vi "Vision Processing.vi"(4 "error in (no error)":errorcluster, 7 "Image Size":T6=enum."320x240") -> ()   [LabVIEW 2014]
doc: "This VI runs in parallel to other tasks. It gets images from the camera, processes them for color or shape and use that information to affect robot behavior."
uses:
  <vilib>/Rock Robotics/WPI/Camera/WPI_CameraImageSize.ctl
  Program Files (x86)/National Instruments/LabVIEW 2014/examples/FRC/roboRIO/Vision/2015 Vision Example/Vision Support Code/Camera Types.ctl
  <vilib>/Rock Robotics/WPI/Camera/WPI_CameraWhite Balance Values.ctl
  <vilib>/Rock Robotics/WPI/Camera/WPI_CameraExposure Values.ctl
  <vilib>/Rock Robotics/WPI/Camera/WPI_CameraFrameRate.ctl
  <vilib>/vision/Pattern Matching.llb/IMAQ Match Range Setting.ctl
  <vilib>/vision/Pattern Matching.llb/IMAQ Curve Parameters.ctl
  Robot Global Data.vi
  Global 2.vi
  <vilib>/vision/NI_Vision_Development_Module.lvlib
panel:
  out "Scale":dbl
  out "LeftSide":dbl
  out "RightSide":dbl
  out "Detected Totes":T1(array[cluster]) {"Normalized Rect"."Numeric 5" format="%#_2g"; "Normalized Rect"."Numeric 3" format="%#_2g"; "Normalized Rect"."Numeric 2" format="%#_2g"; "Normalized Rect"."Numeric" format="%#_2g"}
  out "Sorted Scores":T2(array[cluster]) {"Correlation" format="%#_3g"; "Scale %" format="%#_3g"; "Score" format="%#_3g"}
  in  "Score Threshold":dbl=75.0
  in  "Annotate":bool=TRUE
  in  "Camera Type":T3=enum."MS HD3000 square"
  out "ms to process":u32
  out "Camera Image":T4(plugin-control)
  out "Template 2":T4(plugin-control)
  out "Masked":T4(plugin-control)
  in  "Tote Color":T5={"Hue"={23.67058792990901, 48.923317529462665}, "Sat"={66.78571428571429, 255.0}, "Val"={48.571428571428584, 255.0}} {"Hue" scale=0.0..255.0 scale format="%#_3g"}
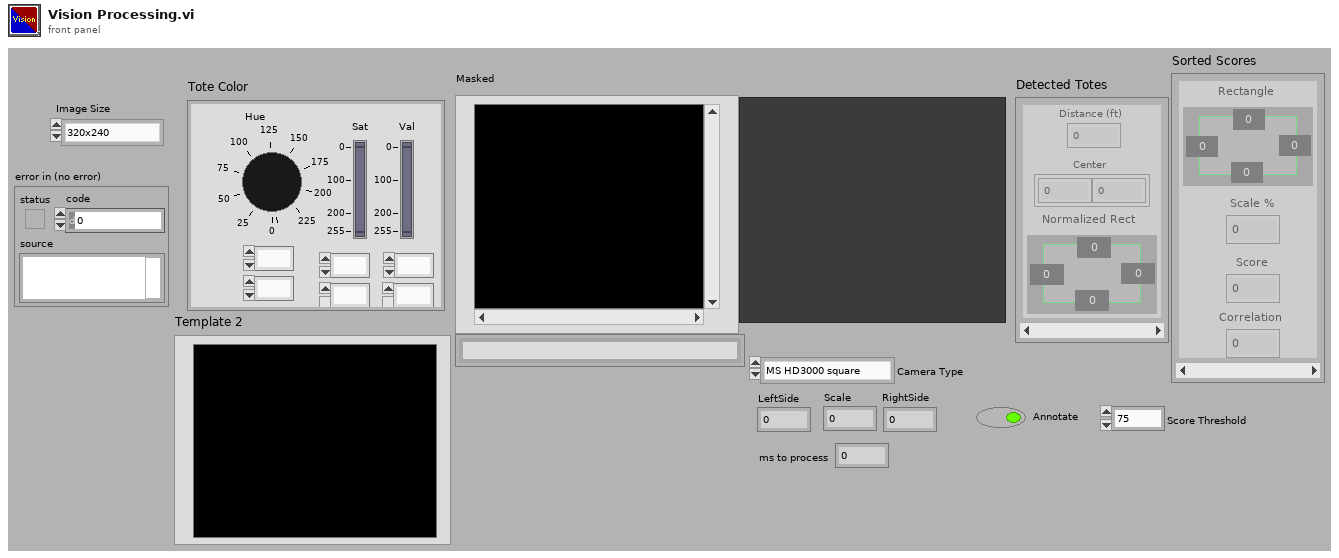
[diagram p1: front panel]
types:
  T1 = cluster{"Distance (ft)":dbl, "Center":cluster{dbl, dbl}, "Normalized Rect":cluster{"Numeric":dbl, "Numeric 2":dbl, "Numeric 3":dbl, "Numeric 5":dbl}}[]
  T2 = cluster{"Rectangle":cluster{"Numeric":dbl, "Numeric 2":dbl, "Numeric 3":dbl, "Numeric 5":dbl}, "Scale %":dbl, "Score":dbl, "Correlation":dbl}[]
  T3 = typedef "Camera Types.ctl" = enum16{"206", "1011", "1013", "MS HD3000 square", "MS HD3000 640x480"}
  T4 = typedef "IMAQ Image.ctl" = refnum<image>
  T5 = cluster{"Hue":cluster{dbl, dbl}, "Sat":cluster{dbl, dbl}, "Val":cluster{dbl, dbl}}
  T6 = typedef "WPI_CameraImageSize.ctl" = enum16{"640x480", "320x240", "160x120", "Custom"}
  T7 = cluster{"Rotation":bool, "Scale":bool, "Occlusion":bool, "Reserved":bool, "Reserved":bool, "Reserved":bool}
  T8 = typedef "IMAQ Curve Parameters.ctl" = cluster{"Extraction Mode":u32, "Edge Threshold":i32, "Edge Filter Size":u32, "Min Length":i32, "Row Search Step Size":i32, "Col Search Step Size":i32, "Max Endpoint Gap":i32, "Closed":bool, "Subpixel":bool}
  T9 = typedef "IMAQ Match Range Setting.ctl" = cluster{"Match Constraints":u32, "Min":dbl, "Max":dbl}
  T10 = typedef "Image Type" = u32
  T11 = typedef "Particle Parameters" = i32
  T12 = typedef "WPI_CameraFrameRate.ctl" = u32
  T13 = typedef "WPI_CameraExposure Values.ctl" = enum16{"Auto", "Flicker-free 50 Hz", "Flicker-free 60 Hz", "Hold current", "Custom"}
  T14 = typedef "WPI_CameraWhite Balance Values.ctl" = enum16{"Auto", "Fixed indoor", "Fixed outdoor 1", "Fixed outdoor 2", "Fixed fluorescent 1", "Fixed fluorescent 2", "Hold current", "Custom"}
  T15 = typedef "WPI_CameraDevRef.ctl" = cluster{"Camera Address":string, "CameraStatus":errorcluster}
  T16 = cluster{"[0]":dbl, "[1]":dbl, "[2]":dbl, "[3]":dbl}
  T17 = cluster{"[0]":dbl, "[1]":dbl, "[2]":dbl, "[3]":dbl, "[4]":dbl}
  T18 = typedef "ROI Descriptor" = cluster{"Global Rectangle":i32[], "Contours":cluster{"ID":enum32{"External", "Internal"}, "Type":u32, "Coordinates":i32[]}[]}
  T19 = typedef "IMAQ GM Match Report.ctl" = cluster{"Position":cluster{"x":sgl, "y":sgl}, "Angle":sgl, "Scale":sgl, "Score":sgl, "Bounding Box":cluster{"x":sgl, "y":sgl}[], "Contrast Reversed":bool, "Occlusion %":sgl, "Template Target Curve Score":sgl, "Target Template Curve Score":sgl, "Correlation Score":sgl}
  T20 = cluster{cluster{"[0]":dbl, "[1]":dbl, "[2]":dbl, "[3]":dbl}, "Position":cluster{"x":sgl, "y":sgl}, "Bounding Box":cluster{"x":sgl, "y":sgl}[], "Scale":sgl, "Score":sgl, "Correlation Score":sgl}
  T21 = cluster{"Rectangle":cluster{"Numeric":dbl, "Numeric 2":dbl, "Numeric 3":dbl, "Numeric 5":dbl}, "Scale":dbl, "Score":dbl, "Correlation":dbl}[]
  T22 = cluster{"Sorted Scores[0]":cluster{"Rectangle":cluster{"Numeric":dbl, "Numeric 2":dbl, "Numeric 3":dbl, "Numeric 5":dbl}, "Scale":dbl, "Score":dbl, "Correlation":dbl}, "Sorted Scores[1]":cluster{"Rectangle":cluster{"Numeric":dbl, "Numeric 2":dbl, "Numeric 3":dbl, "Numeric 5":dbl}, "Scale":dbl, "Score":dbl, "Correlation":dbl}, "Sorted Scores[2]":cluster{"Rectangle":cluster{"Numeric":dbl, "Numeric 2":dbl, "Numeric 3":dbl, "Numeric 5":dbl}, "Scale":dbl, "Score":dbl, "Correlation":dbl}, "Sorted Scores[3]":cluster{"Rectangle":cluster{"Numeric":dbl, "Numeric 2":dbl, "Numeric 3":dbl, "Numeric 5":dbl}, "Scale":dbl, "Score":dbl, "Correlation":dbl}, "Sorted Scores[4]":cluster{"Rectangle":cluster{"Numeric":dbl, "Numeric 2":dbl, "Numeric 3":dbl, "Numeric 5":dbl}, "Scale":dbl, "Score":dbl, "Correlation":dbl}, "Sorted Scores[5]":cluster{"Rectangle":cluster{"Numeric":dbl, "Numeric 2":dbl, "Numeric 3":dbl, "Numeric 5":dbl}, "Scale":dbl, "Score":dbl, "Correlation":dbl}, "Sorted Scores[6]":cluster{"Rectangle":cluster{"Numeric":dbl, "Numeric 2":dbl, "Numeric 3":dbl, "Numeric 5":dbl}, "Scale":dbl, "Score":dbl, "Correlation":dbl}, "Sorted Scores[7]":cluster{"Rectangle":cluster{"Numeric":dbl, "Numeric 2":dbl, "Numeric 3":dbl, "Numeric 5":dbl}, "Scale":dbl, "Score":dbl, "Correlation":dbl}, "Sorted Scores[8]":cluster{"Rectangle":cluster{"Numeric":dbl, "Numeric 2":dbl, "Numeric 3":dbl, "Numeric 5":dbl}, "Scale":dbl, "Score":dbl, "Correlation":dbl}}
  T23 = cluster{"Rectangle":cluster{"Numeric":dbl, "Numeric 2":dbl, "Numeric 3":dbl, "Numeric 5":dbl}, "Scale":dbl, "Score":dbl, "Correlation":dbl}
  T24 = cluster{"Numeric":dbl, "Numeric 2":dbl, "Numeric 3":dbl, "Numeric 5":dbl}
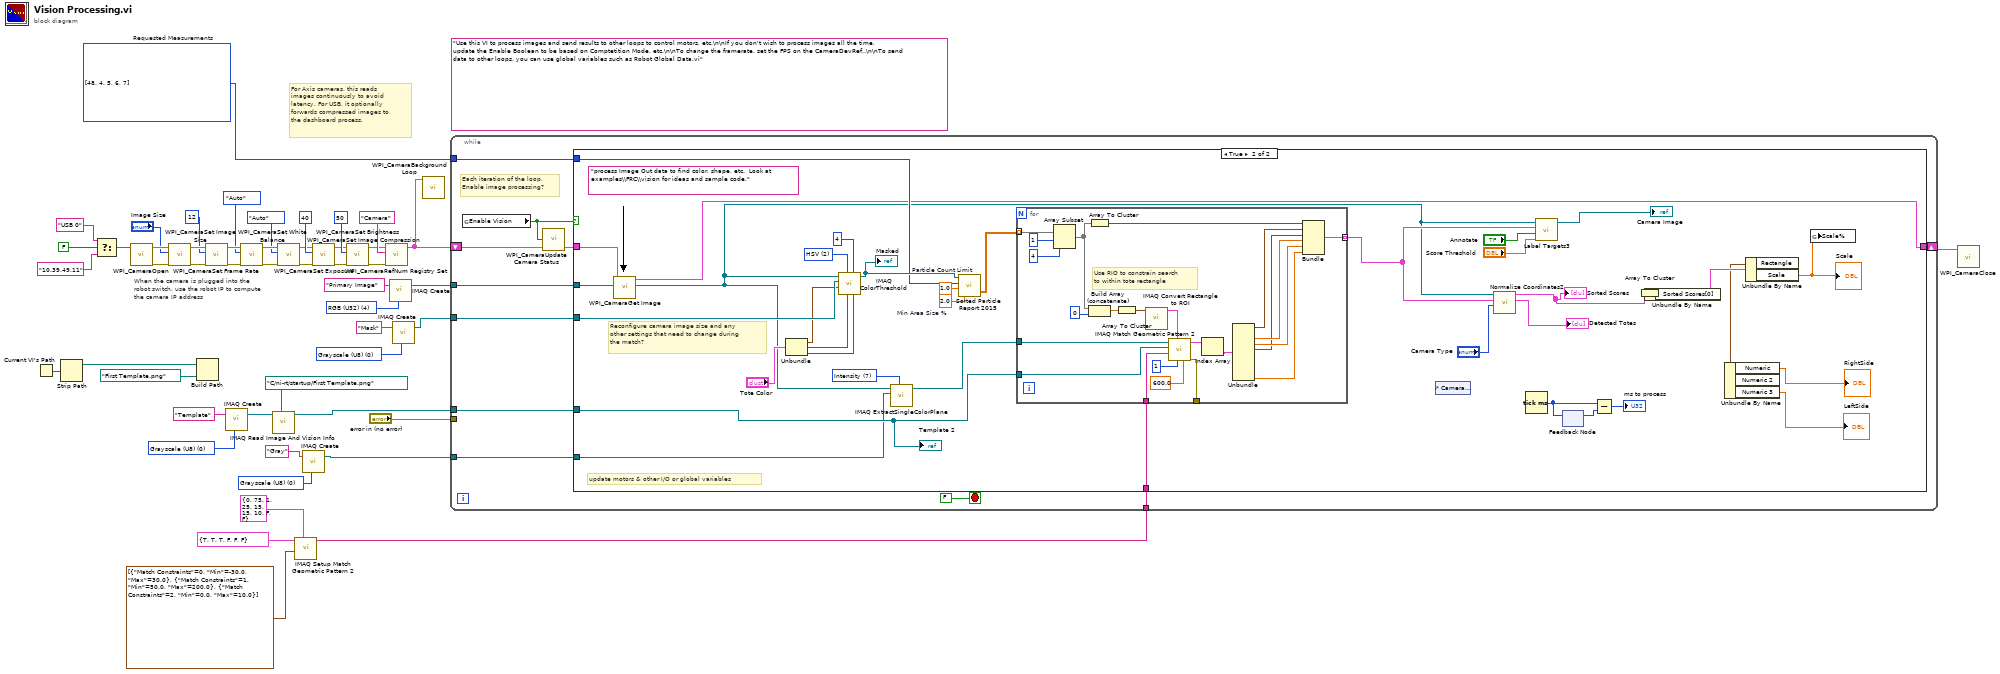
[diagram p0: block diagram]
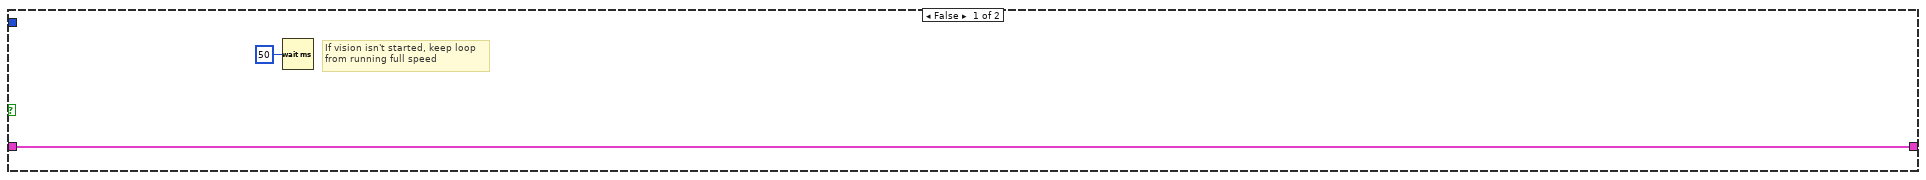
[diagram p2: hidden frame]
diagram:
  w11 = T10 0 items=["Grayscale (U8)", "Grayscale (I16)", "Grayscale (SGL)", "Complex (CSG)", "RGB (U32)", "HSL (U32)", "RGB (U64)", "Grayscale (U16)"] ("Image Type")
  w15 = T10 0 items=["Grayscale (U8)", "Grayscale (I16)", "Grayscale (SGL)", "Complex (CSG)", "RGB (U32)", "HSL (U32)", "RGB (U64)", "Grayscale (U16)"] ("Image Type")
  w16 = T11[] [48, 4, 5, 6, 7] items=["Center of Mass X", "Center of Mass Y", "First Pixel X", "First Pixel Y", "Bounding Rect Left", "Bounding Rect Top", "Bounding Rect Right", "Bounding Rect Bottom", "Max Feret Diameter Start X", "Max Feret Diameter Start Y", "Max Feret Diameter End X", "Max Feret Diameter End Y", "Max Horiz. Segment Length Left", "Max Horiz. Segment Length Right", "Max Horiz. Segment Length Row", "-", "Bounding Rect Width", "Bounding Rect Height", "Bounding Rect Diagonal", "Perimeter", "Convex Hull Perimeter", "Holes' Perimeter", "Max Feret Diameter", "Equivalent Ellipse Major Axis", "Equivalent Ellipse Minor Axis", "Equivalent Ellipse Minor Axis (Feret)", "Equivalent Rect Long Side", "Equivalent Rect Short Side", "Equivalent Rect Diagonal", "Equivalent Rect Short Side (Feret)", "Average Horiz. Segment Length", "Average Vert. Segment Length", "Hydraulic Radius", "Waddel Disk Diameter", "-", "Area", "Holes' Area", "Particle & Holes' Area", "Convex Hull Area", "Image Area", "-", "Number of Holes", "Number of Horiz. Segments", "Number of Vert. Segments", "-", "Orientation", "Max Feret Diameter Orientation", "-", "% Area/Image Area", "% Area/(Particle & Holes' Area)", "Ratio of Equivalent Ellipse Axes", "Ratio of Equivalent Rect Sides", "-", "Elongation Factor", "Compactness Factor", "Heywood Circularity Factor", "Type Factor", "-", "Sum X", "Sum Y", "Sum XX", "Sum XY", "Sum YY", "Sum XXX", "Sum XXY", "Sum XYY", "Sum YYY", "-", "Moment of Inertia XX", "Moment of Inertia XY", "Moment of Inertia YY", "Moment of Inertia XXX", "Moment of Inertia XXY", "Moment of Inertia XYY", "Moment of Inertia YYY", "Norm. Moment of Inertia XX", "Norm. Moment of Inertia XY", "Norm. Moment of Inertia YY", "Norm. Moment of Inertia XXX", "Norm. Moment of Inertia XXY", "Norm. Moment of Inertia XYY", "Norm. Moment of Inertia YYY", "Hu Moment 1", "Hu Moment 2", "Hu Moment 3", "Hu Moment 4", "Hu Moment 5", "Hu Moment 6", "Hu Moment 7"]  # Requested Measurements
  w19 = T10 0 items=["Grayscale (U8)", "Grayscale (I16)", "Grayscale (SGL)", "Complex (CSG)", "RGB (U32)", "HSL (U32)", "RGB (U64)", "Grayscale (U16)"] ("Image Type")
  (unwired) "Use this VI to process images and send results to other loops to control motors, etc.\n\nIf you don't wish to process images all the time, update the Enable Boolean to be based on Comptetition Mode, etc.\n\nTo change the framerate, set the FPS on the CameraDevRef..\n\nTo send data to other loops, you can use global variables such as Robot Global Data.vi"
  w50 = T10 4 items=["Grayscale (U8)", "Grayscale (I16)", "Grayscale (SGL)", "Complex (CSG)", "RGB (U32)", "HSL (U32)", "RGB (U64)"] ("Image Type")
  # "When the camera is plugged into the\nrobot switch, use the robot IP to compute\nthe camera IP address"
  # "For Axis cameras, this reads\nimages continuously to avoid\nlatency. For USB, it optionally\nforwards compressed images to\nthe dashboard process."
  n1 = Current VI's Path() -> (path=w3:path)
  n2 = Strip Path(path=w3) -> (stripped path=w2:path)  [unwired: 1 out]
  n3 = Select(t="USB 0" ("format string"), s=FALSE ("dot notation? (F)"), f="10.39.49.11" ("format string")) -> (s? t:f=w21:string)
  n4 = call <vilib>:"WPI_CameraOpen.vi"("Camera Address"=w21) -> ("error out"=w38:errorcluster, "CameraDevRef"=w39:T15)  [unwired: 1 in, 8 out]
  n5 = call <vilib>:"WPI_CameraSet Image Size.vi"("error in (no error)"=w38, "Image Size"="Image Size", "CameraDevRef"=w39) -> ("error out"=w37:errorcluster, "CameraDevRef Out"=w40:T15)  [unwired: 1 in, 6 out]
  n6 = Build Path(base path=w2, name or relative path=path "First Template.png") -> ()  [unwired: 1 out]
  n7 = call <vilib>:"WPI_CameraSet Frame Rate.vi"("error in (no error)"=w37, "Frame Rate (fps)"=T12 12, "CameraDevRef"=w40) -> ("error out"=w36:errorcluster, "CameraDevRef Out"=w42:T15)  [unwired: 7 out]
  n8 = call "IMAQ Create"("Image Name"="Template", "Image Type"=w15) -> ("New Image"=w13:T4)  [unwired: 2 in, 2 out]
  n9 = call <vilib>:"WPI_CameraSet White Balance.vi"("error in (no error)"=w36, "White Balance"=WPI_CameraWhite_Balance_Values."Auto", "CameraDevRef"=w42) -> ("error out"=w35:errorcluster, "CameraDevRef Out"=w41:T15)  [unwired: 1 in, 6 out]
  n10 = call "IMAQ Read Image And Vision Info"("File Path"=path "C:/ni-rt/startup/First Template.png", "Image"=w13) -> ("Image Out"=w12:T4)  [unwired: 2 in, 7 out]
  n11 = call <vilib>:"WPI_CameraSet Exposure.vi"("error in (no error)"=w35, "Exposure"=WPI_CameraExposure_Values."Auto", "CameraDevRef"=w41) -> ("error out"=w34:errorcluster, "CameraDevRef Out"=w44:T15)  [unwired: 1 in, 6 out]
  n12 = call "IMAQ Setup Match Geometric Pattern 2"("Curve Parameters"=T8 {"Extraction Mode"=0, "Edge Threshold"=75, "Edge Filter Size"=1, "Min Length"=25, "Row Search Step Size"=15, "Col Search Step Size"=15, "Max Endpoint Gap"=10, "Closed"=FALSE, "Subpixel"=FALSE}, "Range Settings"=T9[] [{"Match Constraints"=0, "Min"=-30.0, "Max"=30.0}, {"Match Constraints"=1, "Min"=50.0, "Max"=200.0}, {"Match Constraints"=2, "Min"=0.0, "Max"=10.0}], "Match Mode"=T7 {"Rotation"=TRUE, "Scale"=TRUE, "Occlusion"=TRUE, "Reserved"=FALSE, "Reserved"=FALSE, "Reserved"=FALSE}) -> ("Match Geometric Pattern 2 Setup Data"=w5:string)  [unwired: 7 in, 1 out]
  n13 = call "IMAQ Create"("Image Name"="Gray", "Image Type"=w11) -> ("New Image"=w9:T4)  [unwired: 2 in, 2 out]
  n14 = call <vilib>:"WPI_CameraSet Image Compression.vi"("error in (no error)"=w34, "Compression"=40, "CameraDevRef"=w44) -> ("error out"=w33:errorcluster, "CameraDevRef Out"=w43:T15)  [unwired: 7 out]
  n15 = call <vilib>:"WPI_CameraSet Brightness.vi"("error in (no error)"=w33, "Brightness"=50, "CameraDevRef"=w43) -> ("error out"=w31:errorcluster, "CameraDevRef Out"=w32:T15)  [unwired: 7 out]
  n16 = call <vilib>:"WPI_CameraRefNum Registry Set.vi"("error in (no error)"=w31, "refnum name"="Camera", "CameraDevRef"=w32) -> ("CameraDevRef"=w27:T15)  [unwired: 8 out]
  n17 = call "IMAQ Create"("Image Name"="Primary Image", "Image Type"=w50) -> ("New Image"=w48:T4)  [unwired: 2 in, 2 out]
  n18 = call "IMAQ Create"("Image Name"="Mask", "Image Type"=w19) -> ("New Image"=w17:T4)  [unwired: 2 in, 2 out]
  n19 = call <vilib>:"WPI_CameraBackground Loop.vi"("CameraDevRef"=w27) -> ()  [unwired: 11 in]
  n20 = while {
    shift-right: [w51] -> w25
    shift-left: w27 -> [w59]
    tunnel: w48 -> [w60]
    tunnel: "error in (no error)" -> [_]
    tunnel: w17 -> [w56]
    tunnel: w16 -> [w55]
    tunnel: w12 -> [w54]
    tunnel: w9 -> [w53]
    tunnel: w5 -> [w52]
    stop <- FALSE stop-if-true
    # "Each iteration of the loop,\nEnable image processing?"
    n21 = global read "Robot Global Data.vi" "Enable Vision"() -> (w57:bool)
    n22 = call <vilib>:"WPI_CameraUpdate Camera Status.vi"("CameraDevRef In"=w59, "Enable Vision"=w57) -> ("CameraDevRef Out"=w58:T15)  [unwired: 3 in]
    n23 = case shown="True" w57 {
      tunnel: w60 -> [_ w100]
      tunnel: w58 -> [w62 w99]
      tunnel: w56 -> [_ w98]
      tunnel: w55 -> [_ w90]
      tunnel: w54 -> [_ w84]
      tunnel: w53 -> [_ w83]
      tunnel: w52 -> [_ w82]
      tunnel: [w62 w68] -> w51
      frame False {
        # "If vision isn't started, keep loop\nfrom running full speed"
        n24 = Wait (ms)(milliseconds to wait=u32 50) -> ()  [unwired: 1 out]
      }
      frame True {
        w86 = 7 items=["Red", "Green", "Blue", "Hue", "Saturation", "Luminance", "Value", "Intensity"] ("Color Plane")
        w88 = 2.0  # Min Area Size %
        w89 = 1.0  # Particle Count Limit
        w93 = u16 2 items=["RGB", "HSL", "HSV", "HSI"] ("Color Mode")
        (unwired) "process Image Out data to find color, shape, etc.  Look at examples\\FRC\\vision for ideas and sample code."
        # "update motors & other I/O or global variables"
        # "Reconfigure camera image size and any\nother settings that need to change during\nthe match?"
        n25 = call <vilib>:"WPI_CameraGet Image.vi"("Image"=w100, "CameraDevRef"=w99) -> ("Image Out"=w67:T4, "CameraDevRef Out"=w68:T15)  [unwired: 1 in, 7 out]
        n26 = Unbundle("Tote Color") -> ("Hue"=w96:cluster{dbl, dbl}, "Sat"=w95:cluster{dbl, dbl}, "Val"=w94:cluster{dbl, dbl})
        n27 = call "IMAQ ColorThreshold"("Blue or Luma or Val or Inten Range"=w94, "Replace Value"=4, "Green or Sat Range"=w95, "Color Mode"=w93, "Red or Hue Range"=w96, "Image Dst"=w98, "Image Src"=w67) -> ("Image Dst Out"=w91:T4)  [unwired: 3 in, 1 out]
        "Masked" <- w91
        n28 = call "IMAQ ExtractSingleColorPlane"("Color Plane"=w86, "Image Dst"=w83, "Image Src"=w67) -> ("Image Dst Out"=w85:T4)  [unwired: 7 in, 1 out]
        n29 = call "Sorted Particle Report 2015.vi"("Min Area Size %"=w88, "Particle Count Limit"=w89, "Pixel Measurements"=w90, "Image in"=w91) -> ("Sorted Data"=w87:dbl[][])  [unwired: 1 out]
        n30 = for {
          tunnel: w87 -> [w121] mode=indexing
          tunnel: [w120] -> w70 mode=indexing
          tunnel: w85 -> [w111]
          tunnel: w82 -> [w113]
          tunnel: w84 -> [w103]
          tunnel: [w102] -> _
          # "Use RIO to constrain search\nto within tote rectangle"
          n31 = Array Subset(array=w121, index=1, length=4) -> (w114:dbl[])
          n32 = Array To Cluster(array=w114) -> (cluster=w115:T16)
          n33 = Build Array (concatenate)(w114, 0 ("length")) -> (w118:dbl[])
          n34 = Array To Cluster(array=w118) -> (cluster=w117:T17)
          n35 = call "IMAQ Convert Rectangle to ROI"("Rectangle"=w117) -> ("ROI Descriptor"=w116:T18)  [unwired: 8 in, 1 out]
          n36 = call "IMAQ Match Geometric Pattern 2"("Minimum Match Score"=sgl 600.0, "Number of Matches Requested"=1 ("Minimum Match Score"), "ROI Descriptor"=w116, "Match Geometric Pattern 2 Setup Data"=w113, "Template Image"=w103, "Image"=w111) -> ("error out"=w102:errorcluster, "Matches (pixel)"=w109:T19[])  [unwired: 2 in, 2 out]
          n37 = Index Array(array=w109) -> (element=w108:T19)  [unwired: 1 in]
          n38 = Unbundle(w108) -> ("Position"=w107:cluster{"x":sgl, "y":sgl}, "Scale"=w106:sgl, "Score"=w105:sgl, "Bounding Box"=w101:cluster{"x":sgl, "y":sgl}[], "Correlation Score"=w104:sgl)  [unwired: 5 out]
          n39 = Bundle(w115, "Position"=w107, "Bounding Box"=w101, "Scale"=w106, "Score"=w105, "Correlation Score"=w104) -> (w120:T20)  [unwired: 1 in]
        }
        n40 = control-ref of="Camera Type"() -> ()  [unwired: 1 out]
        n41 = call "Normalize Coordinates2.vi"("Camera Type"="Camera Type", "Targets"=w70, "Image in"=w67) -> ("Found Totes"=→"Detected Totes":T1, "Sorted Scores"=w74:T21)  [unwired: 7 in]
        "Sorted Scores" <- w74
        n42 = Tick Count (ms)() -> (millisecond timer value=w80:u32)
        n43 = call "Label Targets3.vi"("Score Threshold"="Score Threshold", "Annotate"="Annotate", "Targets"=w70, "Image in"=w67) -> ("Image out"=→"Camera Image":T4)  [unwired: 7 in]
        n44 = feedback #1() -> (w81:u32)  [unwired: 1 in]
        n45 = feedback-in #1(w80) -> ()
        n46 = Subtract(x=w80, y=w81) -> (x-y=→"ms to process":u32)
        n47 = Array To Cluster(array=w74) -> (cluster=w73:T22)
        n48 = Unbundle By Name(w73) -> ("Sorted Scores[0]"=w72:T23)
        n49 = Unbundle By Name(w72) -> ("Rectangle"=w66:T24, "Scale"=w69:dbl)
        "Scale" <- w69
        n50 = Unbundle By Name(w66) -> ("Numeric"=→"RightSide":dbl, "Numeric 3"=→"LeftSide":dbl)  [unwired: 1 out]
        n51 = global write "Global 2.vi" "Scale%"(w69) -> ()
        "Template 2" <- w84
      }
    }
  }
  n52 = call <vilib>:"WPI_CameraClose.vi"("CameraDevRef"=w25) -> ()  [unwired: 1 in, 10 out]
